vi "ReadData7.vi"() -> ()   [LabVIEW 2013]
uses:
  <vilib>/Utility/file.llb/Read From Spreadsheet File (DBL).vi
  <vilib>/Analysis/NI_AALPro.lvlib
  <vilib>/Analysis/NI_AALBase.lvlib
panel:
  in  "# skip":i32=100
  out "Residual (V)":dbl=-0.2760035874861321 format="%#_3g"
  in  "1st sweep":i32=400
  in  "# of sweeps":i32=1000
  out "Mean Error":dbl=0.00024772361252328154 format="%#_2g"
  out "Mean Area":dbl=0.0012416466800689867 format="%#_4g"
  out "Spectrum #":i32=999
  out "Chars":i32=1282716
  out "Fcen":dbl=213.0 format="%#_13g"
  in  "Fmin":dbl=212.8 format="%#_13g"
  in  "Fmax":dbl=213.2 format="%#_13g"
  out "# Data points":i32=81
  out "Peak Area (V-MHz)":dbl=0.000769766287548759 format="%#_3g"
  in  "Offset V":dbl=0.118 format="%#_3g"
  out "RMS Fit Error (V)":dbl=0.29222500267003976 format="%#_2g"
  in  "Start sigma (V)":dbl=0.01 format="%#_13g"
  in  "Start offset (V)":dbl format="%#_13g"
  out "FWHM (MHz)":dbl=0.0235 format="%#_3g"
  out "Center Freq (MHz)":dbl=213.2
  out "Amplitude (V)":dbl=0.030717018909899838 format="%#_3g"
  out "NMR Graph + Fit":cluster{dbl, dbl}[](graph)=[{212.8, -0.46521245828698476}, {212.805, -0.451738042269188}, {212.81, -0.4361992213570638}, {212.815, -0.423063070077864}, {212.82000000000002, -0.4129858731924357}, {212.82500000000002, -0.39950200222469395}, {212.83, -0.3896972191323693}, {212.835, -0.37960778642936577}, {212.84, -0.3704715239154619}, {212.845, -0.3613756395995548}, {212.85000000000002, -0.3542806451612908}, {212.85500000000002, -0.34573826473859853}, {212.86, -0.3389151279199112}, {212.865, -0.3356645161290327}, {212.87, -0.32928698553948893}, {212.875, -0.3245533926585096}, {212.88, -0.3195674082313677}, {212.88500000000002, -0.31636484983314794}, {212.89000000000001, -0.31329766407119025}, {212.895, -0.30928097886540584}, {212.9, -0.3076335928809786}, {212.905, -0.3051696329254729}, {212.91, -0.3036011123470524}, {212.915, -0.3027078976640709}, {212.92000000000002, -0.3008886540600665}, {212.925, -0.30022525027808694}, {212.93, -0.30038031145717464}, {212.935, -0.29949098998887647}, {212.94, -0.2997696329254728}, {212.945, -0.2997037819799777}, {212.95, -0.3008530589543934}, {212.955, -0.30116340378198003}, {212.96, -0.3008441601779759}, {212.965, -0.30301490545050047}, {212.97, -0.30069076751946616}, {212.975, -0.3028248053392658}, {212.98, -0.303430144605117}, {212.985, -0.30305194660734136}, {212.99, -0.30589265850945535}, {212.995, -0.30519688542825396}, {213.0, -0.30662758620689673}, {213.005, -0.30504037819799745}, {213.01, -0.3073824249165735}, {213.015, -0.30678731924360375}, {213.02, -0.3061101223581758}, {213.025, -0.30651223581757503}, {213.03, -0.3057032258064513}, {213.035, -0.3055011123470525}, {213.04, -0.3034794215795326}, {213.045, -0.3025264738598445}, {213.05, -0.29928598442714127}, {213.055, -0.2987539488320353}, {213.06, -0.2956502780867632}, {213.065, -0.2924911012235821}, {213.07, -0.28922858731924417}, {213.075, -0.2846795328142374}, {213.07999999999998, -0.2807577308120136}, {213.085, -0.2763669632925469}, {213.09, -0.2720147942157951}, {213.095, -0.26477352614015554}, {213.1, -0.2591063403781981}, {213.105, -0.250758954393771}, {213.10999999999999, -0.24276573971078985}, {213.11499999999998, -0.23413014460511672}, {213.12, -0.2249777530589542}, {213.125, -0.21574538375973307}, {213.13, -0.20545450500556167}, {213.135, -0.19439221357063405}, {213.14, -0.18102413793103433}, {213.14499999999998, -0.16831835372636259}, {213.14999999999998, -0.15441256952169063}, {213.155, -0.14002936596218032}, {213.16, -0.12397185761957694}, {213.165, -0.10871190211345938}, {213.17, -0.09141713014460523}, {213.17499999999998, -0.07229299221357056}, {213.17999999999998, -0.05475406006674076}, {213.185, -0.033457730812013316}, {213.19, -0.01384126807563961}, {213.195, 0.007918464961067835}, {213.2, 0.030717018909899838}]
  out "File size (bytes)":i32=1284000
  out "File name":string="C:\\Documents and Settings\\Patrick McGaughey\\Desktop\\rssmt\\NMR3489070215.xls"
  # "Gaussian Fit Results"
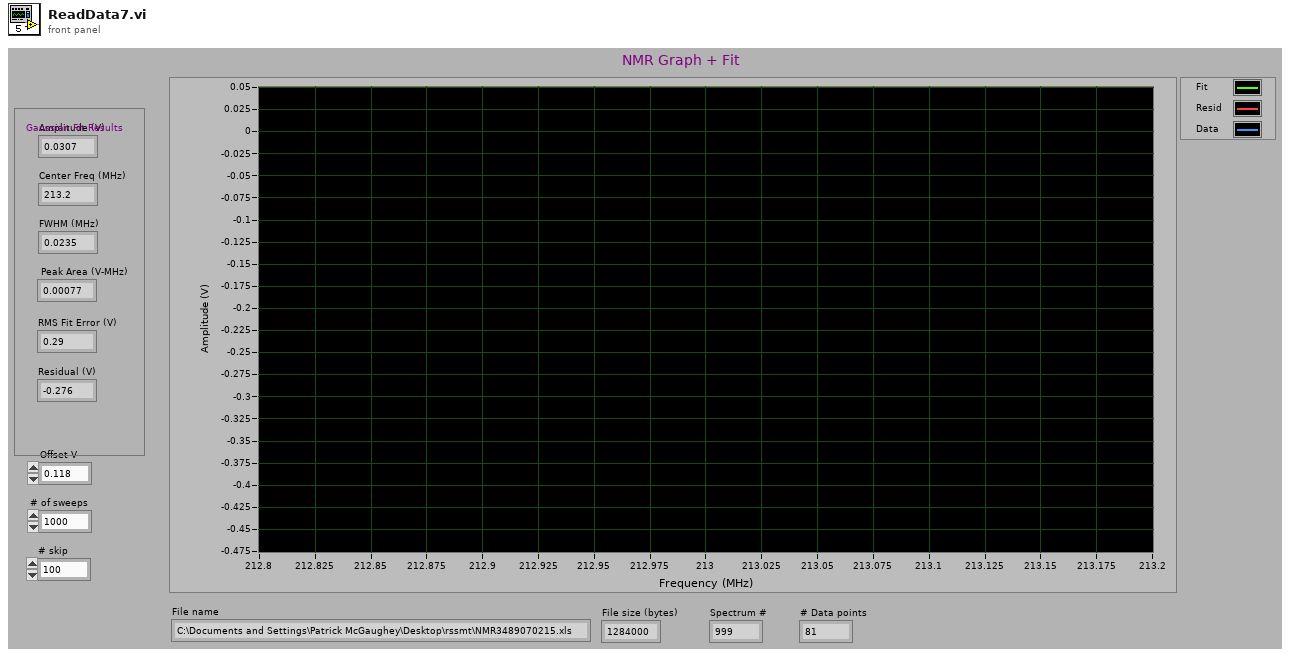
[diagram p1: front panel]
types:
  T1 = cluster{dbl, dbl, "Start sigma (V)":dbl, "Start offset (V)":dbl}
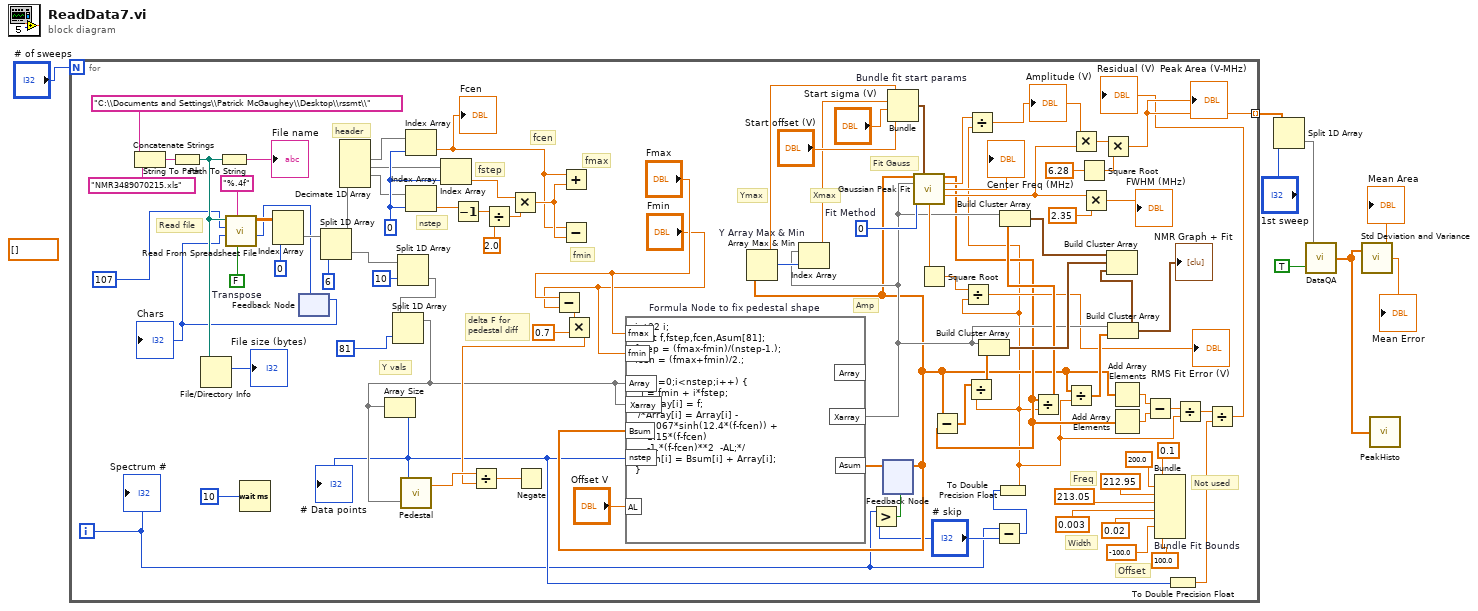
[diagram p0: block diagram]
diagram:
  (unwired) dbl[] []
  n1 = for {
    N: "# of sweeps" -> [_]
    tunnel: [w51] -> w3 mode=indexing
    i -> [w11]
    w62 = 0
    w88 = 0  # Fit Method
    w96 = FALSE  # Transpose
    # "Offset"
    # "Width"
    # "Freq"
    # "Not used"
    # "Fit Gauss"
    # "Read file"
    # "header"
    # "nstep"
    # "fstep"
    # "fcen"
    # "fmin"
    # "fmax"
    # "Amp"
    # "delta F for\npedestal diff"
    # "Ymax"
    # "Xmax"
    # "Y vals"
    n2 = Concatenate Strings "Concatenate Strings"("C:\\Documents and Settings\\Patrick McGaughey\\Desktop\\rssmt\\", "NMR3489070215.xls") -> (w99:string)
    n3 = String To Path(string=w99) -> (path=w95:path)
    n4 = File/Directory Info(path=w95) -> (size=→"File size (bytes)":i64)  [unwired: 1 in, 6 out]
    n5 = Path To String(path=w95) -> (string=→"File name":string)
    n6 = Wait (ms)(milliseconds to wait=10) -> ()  [unwired: 1 out]
    n7 = feedback #1() -> (w52:i32)  [unwired: 1 in]
    "Chars" <- w52
    n8 = call-poly <vilib>:"Read From Spreadsheet File.vi"("transpose (no:F)"=w96, "format (%.3f)"="%.4f", "start of read offset (chars.:0)"=w52, "number of rows (all:-1)"=107, "file path (dialog if empty)"=w95) -> ("mark after read (chars.)"=w53:i32, "all rows"=w70:dbl[][])  [unwired: 2 in, 3 out]
    n9 = Index Array "Index Array"(array=w70, index (col)=0) -> (element=w68:dbl[])  [unwired: 1 in]
    n10 = feedback-in #1(w53) -> ()
    n11 = Split 1D Array(array=w68, index=6) -> (first subarray=w71:dbl[], second subarray=w46:dbl[])
    n12 = Decimate 1D Array(w71) -> (w63:dbl[], w61:dbl[], w60:dbl[])  [unwired: 3 out]
    n13 = Split 1D Array(array=w46, index=10) -> (second subarray=w44:dbl[])  [unwired: 1 out]
    n14 = Split 1D Array(array=w44, index=81) -> (first subarray=w42:dbl[])  [unwired: 1 out]
    n15 = Array Size(array=w42) -> (size(s)=w15:i32)
    "# Data points" <- w15
    n16 = call "Pedestal.vi"("Varray"=w42, "ArraySize"=w15) -> ("L-R"=w82:dbl)  [unwired: 1 out]
    n17 = Index Array "Index Array"(array=w63, index=w62) -> (element=w54:dbl)
    "Fcen" <- w54
    n18 = Index Array(array=w60, index=w62) -> (element=w58:dbl)
    n19 = Index Array(array=w61, index=w62) -> (element=w59:dbl)
    n20 = Decrement(x=w58) -> (x-1=w67:dbl)
    n21 = Divide(x=w67, y=2.0) -> (x/y=w65:dbl)
    n22 = Multiply(x=w59, y=w65) -> (x*y=w64:dbl)
    n23 = Subtract(x="Fmax", y="Fmin") -> (x-y=w80:dbl)
    n24 = Add(x=w54, y=w64) -> ()  [unwired: 1 out]
    n25 = Subtract(x=w54, y=w64) -> ()  [unwired: 1 out]
    n26 = Multiply(x=w80, y=0.7) -> (x*y=w79:dbl)
    n27 = Divide(x=w82, y=w79) -> (x/y=w78:dbl)
    n28 = Negate(x=w78) -> ()  [unwired: 1 out]
    n29 = Greater?(x=w11, y="# skip") -> (0:w13:bool)
    n30 = feedback #2() -> (w22:dbl[])  [unwired: 1 in]
    n31 = formula code="int32 i;\nfloat f,fstep,fcen,Asum[81];\nfstep = (fmax-fmin)/(nstep-1.);\nfcen = (fmax+fmin)/2.;\n\nfor (i=0;i<nstep;i++) {\n  f = fmin + i*fstep;\n  Xarray[i] = f;\n /*Array[i] = Array[i] - \n    0.067*sinh(12.4*(f-fcen)) +\n    1.15*(f-fcen)  \n    -1.*(f-fcen)**2  -AL;*/\nAsum[i] = Bsum[i] + Array[i];\n}" "Formula Node to fix pedestal shape"("nstep"=w15, "fmin"="Fmin", "fmax"="Fmax", "AL"="Offset V", "Array"=w42, "Xarray"=w42, "Bsum"=w22) -> ("Xarray"=w36:dbl[], "Asum"=w50:dbl[])  [unwired: 1 out]
    n32 = Array Max & Min "Y Array Max & Min"(array=w22) -> (max value=w87:dbl, max index (indices)=w86:i32)  [unwired: 2 out]
    n33 = Index Array "Index Array"(array=w36, index=w86) -> (element=w76:dbl)
    n34 = feedback-in #2(w50, w13) -> ()
    n35 = Bundle "Bundle fit start params"(w87, w76, "Start sigma (V)"="Start sigma (V)", "Start offset (V)"="Start offset (V)") -> (w91:T1)  [unwired: 1 in]
    n36 = call <vilib>:"Gaussian Peak Fit.vi"("Y"=w22, "initial guess"=w91, "X"=w36, "method"=w88) -> ("Best Gaussian Fit"=w23:dbl[], "amplitude"=w38:dbl, "center"=→"Center Freq (MHz)":dbl, "standard deviation"=w75:dbl, "residue"=w77:dbl)  [unwired: 5 in, 2 out]
    n37 = Square Root(x=w77) -> (sqrt(x)=w34:dbl)
    n38 = Subtract(x=w22, y=w23) -> (x-y=w48:dbl[])
    n39 = Subtract(x=w11, y="# skip") -> (x-y=w10:i32)
    n40 = To Double Precision Float(number=w10) -> (double precision float=w18:dbl)
    n41 = Divide(x=w34, y=w18) -> (x/y=→"RMS Fit Error (V)":dbl)
    n42 = Divide(x=w48, y=w18) -> (x/y=w47:dbl[])
    n43 = Divide(x=w38, y=w18) -> (x/y=w37:dbl)
    "Amplitude (V)" <- w37
    n44 = Build Cluster Array ("Index & Bundle Cluster Array")(w36, w47) -> (w49:cluster{dbl, dbl}[])
    n45 = Divide(x=w23, y=w18) -> (x/y=w39:dbl[])
    n46 = Build Cluster Array ("Index & Bundle Cluster Array")(w36, w39) -> (w57:cluster{dbl, dbl}[])
    n47 = Divide(x=w22, y=w18) -> (x/y=w35:dbl[])
    n48 = Multiply(x=w37, y=w75) -> (x*y=w83:dbl)
    n49 = Square Root(x=6.28) -> (sqrt(x)=w84:dbl)
    n50 = Multiply(x=w75, y=2.35) -> (x*y=→"FWHM (MHz)":dbl)
    n51 = Multiply(x=w83, y=w84) -> (x*y=w51:dbl)
    "Peak Area (V-MHz)" <- w51
    n52 = Build Cluster Array ("Index & Bundle Cluster Array")(w36, w35) -> (w9:cluster{dbl, dbl}[])
    "NMR Graph + Fit" <- w9
    n53 = Build Cluster Array "Build Cluster Array"(w57, w49, w9) -> ()  [unwired: 1 out]
    n54 = Add Array Elements(numeric array=w22) -> (sum=w20:dbl)
    n55 = Add Array Elements(numeric array=w23) -> (sum=w21:dbl)
    n56 = Subtract(x=w20, y=w21) -> (x-y=w19:dbl)
    n57 = Bundle "Bundle Fit Bounds"(0.1, 200.0, 212.95, 213.05, 0.003, 0.02, -100.0, 100.0) -> ()  [unwired: 1 in, 1 out]
    n58 = To Double Precision Float(number=w15) -> (double precision float=w14:dbl)
    n59 = Divide(x=w19, y=w18) -> (x/y=w17:dbl)
    n60 = Divide(x=w17, y=w14) -> (x/y=→"Residual (V)":dbl)
    "Spectrum #" <- w11
  }
  n61 = Split 1D Array(array=w3, index="1st sweep") -> (second subarray=w1:dbl[])  [unwired: 1 out]
  n62 = call "DataQA.vi"("Quality cuts"=TRUE, "Data In"=w1) -> ("Data Out"=w4:dbl[])
  n63 = call <vilib>:"Std Deviation and Variance.vi"("X"=w4) -> ("mean"=→"Mean Area":dbl, "standard deviation"=→"Mean Error":dbl)  [unwired: 1 in, 1 out]
  n64 = call "PeakHisto.vi"("Data Out"=w4) -> ()  [unwired: 1 out]
